vi "Set Force Units.vi"(8 "error in (no error)":errorcluster, 10 "Force Units":T1, 11 "ESM303 in":refnum<class "ESM303.lvclass">) -> (0 "error out":errorcluster, 3 "ESM303 out":refnum<class "ESM303.lvclass">)   [LabVIEW 2018, in "ESM303.lvlib" / "ESM303.lvclass"]
uses:
  ESM303.lvclass
  builds/Force Test Stand/Force Test Stand/Force Test Stand.lvlibp/Custom Controls/Force Units.ctl
  builds/Force Test Stand/Force Test Stand/Force Test Stand.lvlibp/Force Test Stand.lvclass
  C:/Projects/LabVIEW/In-Progress/Jose Rivero-Diaz/builds/Force Test Stand/Force Test Stand/Force Test Stand.lvlibp/Force Test Stand.lvclass
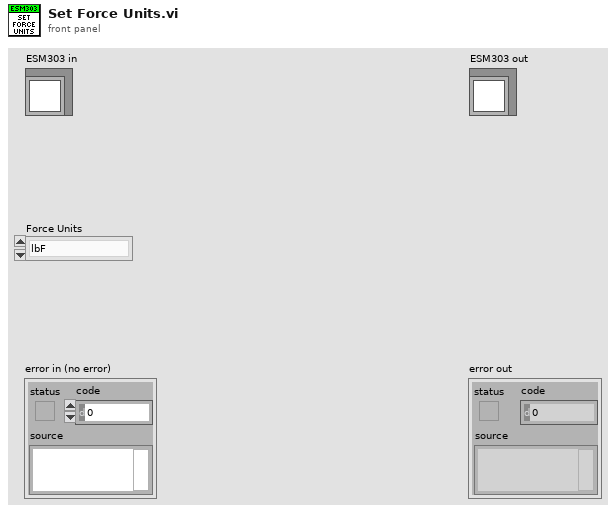
[diagram p1: front panel]
types:
  T1 = typedef "Force Test Stand.lvlibp/Force Test Stand.lvclass/Force Units.ctl" = enum16{"lbF", "ozF", "gF", "kgF", "N", "kN", "mN"}
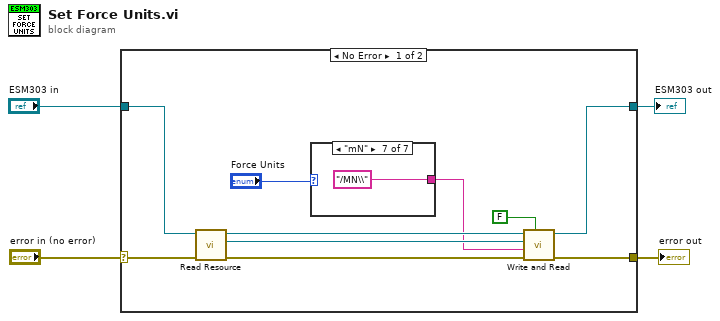
[diagram p0: block diagram]
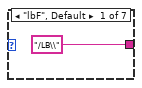
[diagram p2: hidden frame]
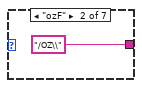
[diagram p3: hidden frame]
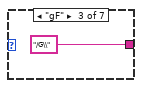
[diagram p4: hidden frame]
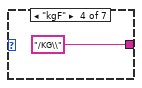
[diagram p5: hidden frame]
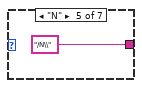
[diagram p6: hidden frame]
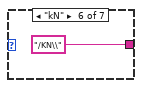
[diagram p7: hidden frame]
diagram:
  n1 = case shown="No Error" "error in (no error)" {
    selector: "error in (no error)" -> [w14 w23]
    tunnel: [w5 w23] -> w3
    tunnel: [w6 w22] -> w2
    tunnel: "ESM303 in" -> [w13 w22]
    frame No Error {
      n2 = call "Read Resource.vi"("error in (no error)"=w14, "Force Test Stand in"=w13) -> ("error out"=w12:errorcluster, "Resource"=w10:refnum<visa-resource-name>, "Force Test Stand out"=w11:refnum<class "ESM303.lvclass">)  [unwired: 7 in]
      n3 = case shown="\"mN\"" "Force Units" {
        tunnel: ["/LB\\" "/OZ\\" "/G\\" "/KG\\" "/N\\" "/KN\\" "/MN\\"] -> w8
        frame "lbF", Default {
        }
        frame "ozF" {
        }
        frame "gF" {
        }
        frame "kgF" {
        }
        frame "N" {
        }
        frame "kN" {
        }
        frame "mN" {
        }
      }
      n4 = call "Write and Read.vi"("Write & Read"=FALSE, "error in (no error)"=w12, "Command"=w8, "VISA Refnum in"=w10, "ESM303 in"=w11) -> ("error out"=w5:errorcluster, "ESM303 out"=w6:refnum<class "ESM303.lvclass">)  [unwired: 4 in, 1 out]
    }
    frame Error {
    }
  }
  "error out" <- w3
  "ESM303 out" <- w2
